vi "FP_recorder 2.vi"() -> ()   [LabVIEW 2013]
uses:
  <userlib>/caLab/Private/Get_PV.vi
panel:
  out "date/time string":string
  out "loop":i32
  out "Cluster":T1
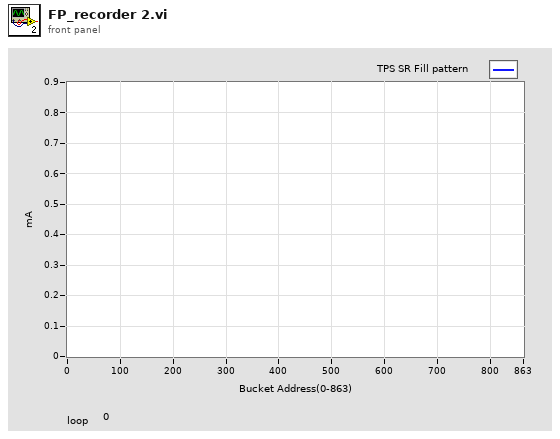
[diagram p1: front panel]
types:
  T1 = cluster{"SR Fill pattern":dbl[], "date/time string":string}
  T2 = typedef "imagedata.ctl" = cluster{"image type":i32, "image depth":i32, "image":u8[], "mask":u8[], "colors":u32[], "Rectangle":cluster{"left":i16, "top":i16, "right":i16, "bottom":i16}}
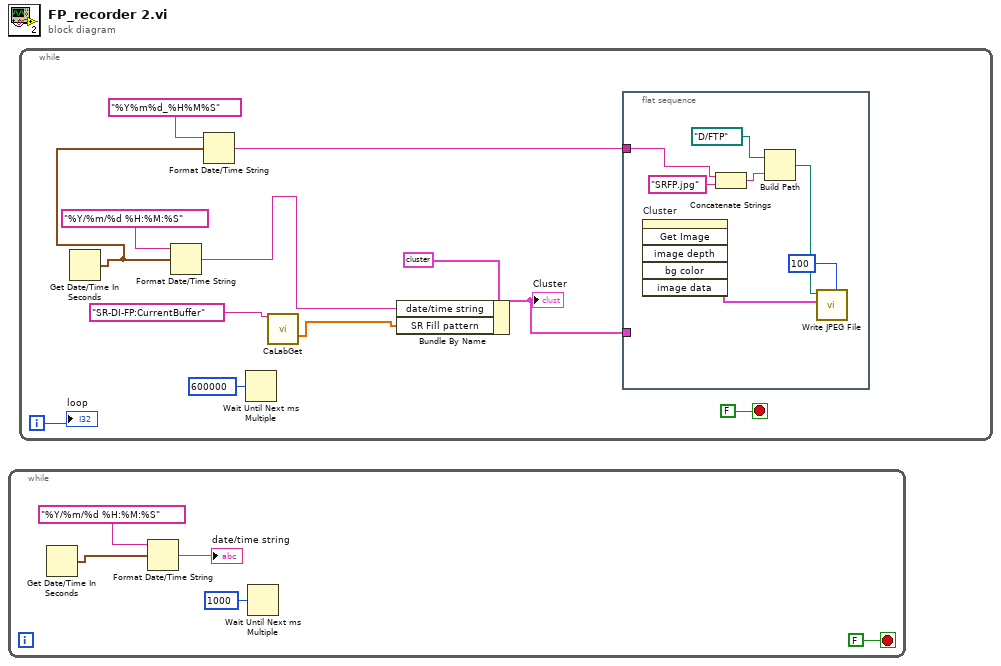
[diagram p0: block diagram]
diagram:
  n1 = while {
    stop <- FALSE stop-if-true
    n2 = Get Date/Time In Seconds() -> (seconds since 1Jan1904=w5:timestamp)
    n3 = Format Date/Time String(time format string (%c)="%Y/%m/%d %H:%M:%S", seconds (now)=w5) -> (date/time string=→"date/time string":string)  [unwired: 1 in]
    n4 = Wait Until Next ms Multiple(millisecond multiple=u32 1000) -> ()  [unwired: 1 out]
  }
  n5 = while {
    i -> [w10]
    stop <- FALSE stop-if-true
    n6 = Get Date/Time In Seconds() -> (seconds since 1Jan1904=w7:timestamp)
    n7 = Format Date/Time String(time format string (%c)="%Y/%m/%d %H:%M:%S", seconds (now)=w7) -> (date/time string=w16:string)  [unwired: 1 in]
    n8 = Format Date/Time String(time format string (%c)="%Y%m%d_%H%M%S", seconds (now)=w7) -> (date/time string=w6:string)  [unwired: 1 in]
    n9 = Wait Until Next ms Multiple(millisecond multiple=u32 600000) -> ()  [unwired: 1 out]
    n10 = call-poly <userlib>:"CaLabGet.vi"("PV Name"="SR-DI-FP:CurrentBuffer") -> ("Value Array (number)"=w17:dbl[])  [unwired: 8 in, 6 out]
    n11 = Bundle By Name(cluster=T1 {"SR Fill pattern"=array[864 elements], "date/time string"=""} ("Cluster"), "date/time string"=w16, "SR Fill pattern"=w17) -> (w11:T1)
    "Cluster" <- w11
    n12 = flat-sequence {
      tunnel: w11 -> [_]
      tunnel: w6 -> [w21]
      frame #0 {
        n13 = invoke on="Cluster" class="Clust (strict)" method="Get Image"() -> ("image data"=w24:T2)  [unwired: 6 in, 5 out]
        n14 = Concatenate Strings(w21, "SRFP.jpg" ("string")) -> (w22:string)
        n15 = Build Path(base path=path "D:/FTP" ("path to JPEG file"), name or relative path=w22) -> (appended path=w19:path)
        n16 = call <vilib>:"Write JPEG File.vi"("quality (80)"=100, "image data"=w24, "path to JPEG file"=w19) -> ()  [unwired: 7 in, 2 out]
      }
    }
    "loop" <- w10
  }
